vi "Main.vi"() -> ()   [LabVIEW 2019]
uses:
  Controls/Save data file action.ctl
  Sub VIs/_Global variables 1.vi
panel:
  in  "stop":bool
  out "Data file\nInitialization":errorcluster
  out "Statues":string
  out "Boolean":bool
  in  "Initialize":bool
  in  "Recording temperature":enum16{"Sample stage", "Mixing chamber"}(ring)
  in  "Heater control":enum16{"Sample stage", "Mixing chamber"}(ring)
  in  "temp step tolerance":dbl=0.02 format="%_3g"
  in  "temperature step":dbl=0.05 format="%_3g"
  in  "Final temperature":dbl format="%_3g"
  in  "Init temperature":dbl format="%_3g"
  in  "Data acquisition field interval (T)":dbl=0.001
  in  "Current source output":dbl=1e-05
  in  "Starting field":dbl format="%_3g"
  in  "field sweeping rate":dbl=0.02 format="%_3g"
  in  "field adjustment rate":dbl=0.05 format="%_3g"
  in  "Stopping field":dbl format="%_3g"
  out "Current source\nInitialization":errorcluster
  out "Magnet Contro Initialization":errorcluster caption="error out"
  out "Sample temp initialization":errorcluster caption="error out"
  out "Temp control initialization":errorcluster caption="error out"
  in  "Start":bool
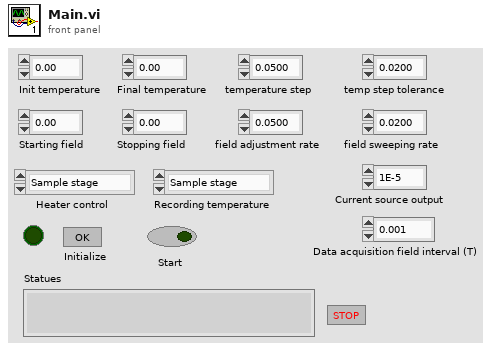
[diagram p1: front panel]
types:
  T1 = typedef "Save data file action.ctl" = enum16{"Create & init file", "Append data", "Close file"}
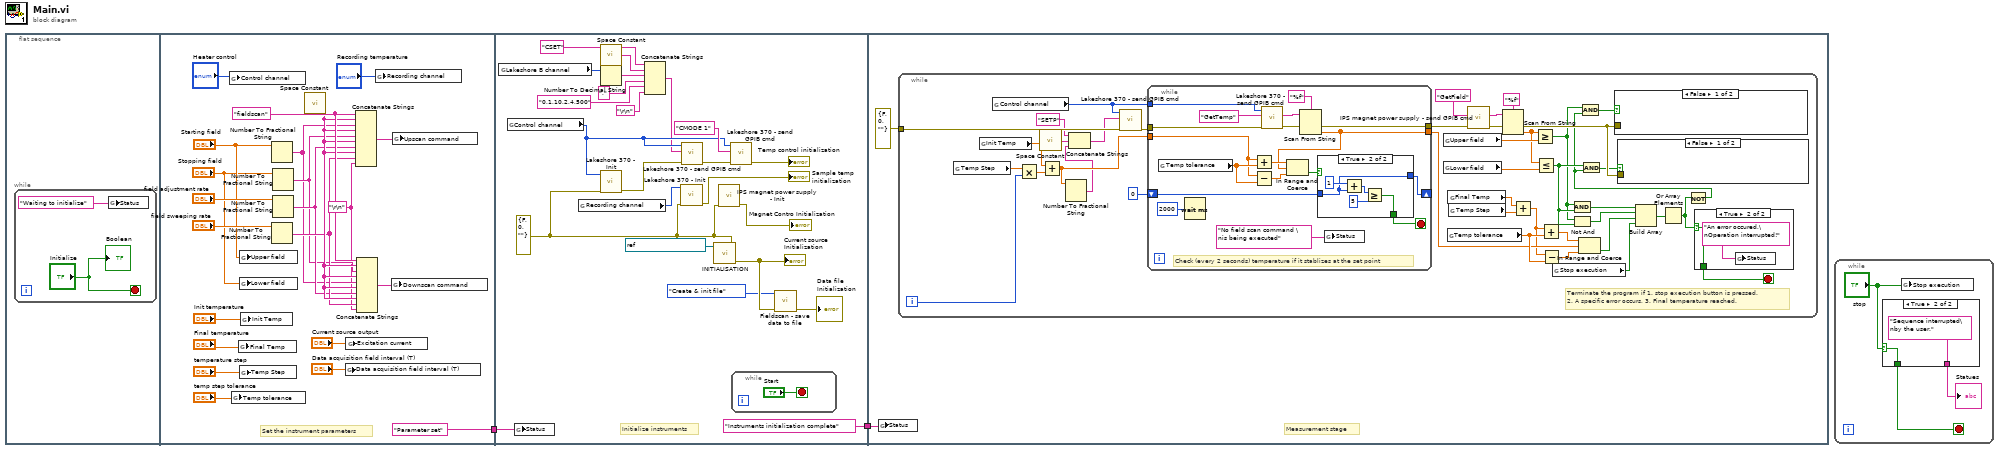
[diagram p0: block diagram]
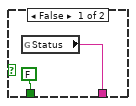
[diagram p2: hidden frame]
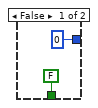
[diagram p4: hidden frame]
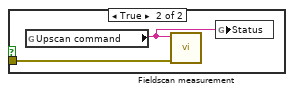
[diagram p5: hidden frame]
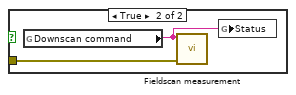
[diagram p6: hidden frame]
diagram:
  n1 = flat-sequence {
    tunnel: ["Parameter set"] -> w2
    tunnel: w2 -> [w43]
    tunnel: ["Instruments initialization complete"] -> w1
    tunnel: w1 -> [w51]
    frame #0 {
      n2 = while {
        stop <- "Initialize" stop-if-true
        n3 = global write "_Global variables 1.vi" "Status"("Waiting to initialize" ("Statues")) -> ()
        "Boolean" <- "Initialize"
      }
    }
    frame #1 {
      w9 = "\r\n"
      w20 = "fieldscan"
      # "Set the instrument parameters"
      n4 = global write "_Global variables 1.vi" "Control channel"("Heater control") -> ()
      n5 = global write "_Global variables 1.vi" "Temp tolerance"("temp step tolerance") -> ()
      n6 = global write "_Global variables 1.vi" "Final Temp"("Final temperature") -> ()
      n7 = global write "_Global variables 1.vi" "Upper field"("Starting field") -> ()
      n8 = global write "_Global variables 1.vi" "Lower field"("Stopping field") -> ()
      n9 = global write "_Global variables 1.vi" "Temp Step"("temperature step") -> ()
      n10 = global write "_Global variables 1.vi" "Init Temp"("Init temperature") -> ()
      n11 = Number To Fractional String(number="Starting field") -> (F-format string=w15:string)  [unwired: 3 in]
      n12 = Number To Fractional String(number="field sweeping rate") -> (F-format string=w18:string)  [unwired: 3 in]
      n13 = Number To Fractional String(number="Stopping field") -> (F-format string=w16:string)  [unwired: 3 in]
      n14 = Number To Fractional String(number="field adjustment rate") -> (F-format string=w17:string)  [unwired: 3 in]
      n15 = call <vilib>:"Space Constant.vi"() -> ("String"=w19:string)
      n16 = global write "_Global variables 1.vi" "Data acquisition field interval (T)"("Data acquisition field interval (T)") -> ()
      n17 = global write "_Global variables 1.vi" "Excitation current"("Current source output") -> ()
      n18 = Concatenate Strings(w20, w19, w15, w19, w16, w19, w17, w19, w18, w9) -> (w10:string)
      n19 = Concatenate Strings(w20, w19, w16, w19, w15, w19, w17, w19, w18, w9) -> (w8:string)
      n20 = global write "_Global variables 1.vi" "Recording channel"("Recording temperature") -> ()
      n21 = global write "_Global variables 1.vi" "Downscan command"(w8) -> ()
      n22 = global write "_Global variables 1.vi" "Upscan command"(w10) -> ()
    }
    frame #2 {
      w46 = errorcluster {"status"=FALSE, "code"=0, "source"=""} ("error in (no error)")
      # "Initialize instruments"
      n23 = global read "_Global variables 1.vi" "Lakeshore B channel"() -> (w34:u8)
      n24 = global read "_Global variables 1.vi" "Control channel"() -> (w35:enum16{"Sample stage", "Mixing chamber"})
      n25 = global write "_Global variables 1.vi" "Status"(w43) -> ()
      n26 = global read "_Global variables 1.vi" "Recording channel"() -> (w44:enum16{"Sample stage", "Mixing chamber"})
      n27 = call <vilib>:"Space Constant.vi"() -> ("String"=w28:string)
      n28 = Number To Decimal String(number=w34) -> (decimal integer string=w32:string)  [unwired: 1 in]
      n29 = call "Lakeshore 370 - Init.vi"("error in (no error)"=w46, "Enum"=w35) -> ("error out"=w45:errorcluster)  [unwired: 8 in, 1 out]
      n30 = Concatenate Strings("CSET" ("Cmd string"), w28, w32, ",", "0,1,10,2,4,500", "\r\n") -> (w29:string)
      n31 = call "Lakeshore 370 - Init.vi"("error in (no error)"=w46, "Enum"=w44) -> ("error out"=→"Sample temp initialization":errorcluster)  [unwired: 8 in, 1 out]
      n32 = call "Lakeshore 370 - send GPIB cmd.vi"("error in (no error)"=w45, "Cmd string"=w29, "Enum"=w35) -> ("error out"=w38:errorcluster)  [unwired: 7 in, 1 out]
      n33 = call "INITIALISATION.vi"("error in (no error)"=w46, "VISAcurrent source"=refnum<visa-resource-name> "GPIB0::12::INSTR" ("Current source")) -> ("error out"=w41:errorcluster)  [unwired: 3 in]
      "Current source\nInitialization" <- w41
      n34 = call "IPS magnet power supply - Init.vi"("error in (no error)"=w46) -> ("error out"=→"Magnet Contro Initialization":errorcluster)  [unwired: 9 in, 1 out]
      n35 = call "Lakeshore 370 - send GPIB cmd.vi"("error in (no error)"=w38, "Cmd string"="CMODE 1", "Enum"=w35) -> ("error out"=→"Temp control initialization":errorcluster)  [unwired: 7 in, 1 out]
      n36 = while {
        stop <- "Start" stop-if-true
      }
      n37 = call "Fieldscan - save data to file.vi"("error in (no error)"=w41, "Action"=Save_data_file_action."Create & init file") -> ("error out"=→"Data file\nInitialization":errorcluster)  [unwired: 8 in, 1 out]
    }
    frame #3 {
      # "Measurement stage"
      n38 = global write "_Global variables 1.vi" "Status"(w51) -> ()
      n39 = while {
        tunnel: errorcluster {"status"=FALSE, "code"=0, "source"=""} ("error in (no error)") -> [w73]
        i -> [w53]
        stop <- w55 stop-if-true
        # "Terminate the program if 1. stop execution button is pressed.\n2. A specific error occurs, 3. Final temperature reached."
        n40 = global read "_Global variables 1.vi" "Temp Step"() -> (w54:dbl)
        n41 = global read "_Global variables 1.vi" "Init Temp"() -> (w71:dbl)
        n42 = global read "_Global variables 1.vi" "Control channel"() -> (w62:enum16{"Sample stage", "Mixing chamber"})
        n43 = Multiply(x=w54, y=w53) -> (x*y=w70:dbl)
        n44 = call <vilib>:"Space Constant.vi"() -> ("String"=w68:string)
        n45 = Add(x=w71, y=w70) -> (x+y=w67:dbl)
        n46 = Number To Fractional String(number=w67) -> (F-format string=w66:string)  [unwired: 3 in]
        n47 = Concatenate Strings("SETP", w68, w66) -> (w65:string)
        n48 = call "Lakeshore 370 - send GPIB cmd.vi"("error in (no error)"=w73, "Cmd string"=w65, "Enum"=w62) -> ("error out"=w72:errorcluster)  [unwired: 7 in, 1 out]
        n49 = while {
          tunnel: w72 -> [w112]
          tunnel: [w107] -> w82
          tunnel: [w105] -> w81
          tunnel: w67 -> [w104]
          shift-right: [w99] -> _
          shift-left: 0 -> [w100]
          tunnel: w62 -> [w98]
          stop <- w101 stop-if-true
          # "Check (every 2 seconds) temperature if it stablizes at the set point"
          n50 = global read "_Global variables 1.vi" "Temp tolerance"() -> (w109:dbl)
          n51 = Wait (ms)(milliseconds to wait=u32 2000) -> ()  [unwired: 1 out]
          n52 = Add(x=w104, y=w109) -> (x+y=w108:dbl)
          n53 = Subtract(x=w104, y=w109) -> (x-y=w110:dbl)
          n54 = call "Lakeshore 370 - send GPIB cmd.vi"("error in (no error)"=w112, "Cmd string"="GetTemp", "Enum"=w98) -> ("error out"=w106:errorcluster, "Response"=w113:string)  [unwired: 7 in]
          n55 = Scan From String(format string="%f", input string=w113, error in=w106) -> (error out=w105:errorcluster, output 1=w107:dbl)  [unwired: 2 in, 2 out]
          n56 = In Range and Coerce(upper limit=w108, x=w107, lower limit=w110) -> (In Range?=w102:bool)  [unwired: 1 out]
          n57 = case shown="True" w102 {
            tunnel: w100 -> [_ w117]
            tunnel: [FALSE w118] -> w101
            tunnel: [0 w117] -> w99
            frame False {
            }
            frame True {
              n58 = Add(x=1, y=w117) -> (x+y=w120:i32)
              n59 = Greater Or Equal?(x=w120, y=5) -> (x >= y?=w118:bool)
            }
          }
          n60 = global write "_Global variables 1.vi" "Status"("No field scan command \nis being executed" ("Downscan command")) -> ()
        }
        n61 = global read "_Global variables 1.vi" "Upper field"() -> (w86:dbl)
        n62 = global read "_Global variables 1.vi" "Lower field"() -> (w84:dbl)
        n63 = global read "_Global variables 1.vi" "Temp tolerance"() -> (w91:dbl)
        n64 = global read "_Global variables 1.vi" "Final Temp"() -> (w75:dbl)
        n65 = global read "_Global variables 1.vi" "Temp Step"() -> (w74:dbl)
        n66 = call "IPS magnet power supply - send GPIB cmd.vi"("error in (no error)"=w81, "Cmd string"="GetField") -> ("error out"=w87:errorcluster, "Response"=w89:string)  [unwired: 8 in]
        n67 = Scan From String(format string="%f", input string=w89, error in=w87) -> (error out=w83:errorcluster, output 1=w85:dbl)  [unwired: 2 in, 2 out]
        n68 = Add(x=w75, y=w74) -> (x+y=w64:dbl)
        n69 = Greater Or Equal?(x=w85, y=w86) -> (x >= y?=w78:bool)
        n70 = Less Or Equal?(x=w85, y=w84) -> (x <= y?=w80:bool)
        n71 = Add(x=w64, y=w91) -> (x+y=w92:dbl)
        n72 = Subtract(x=w64, y=w91) -> (x-y=w93:dbl)
        n73 = global read "_Global variables 1.vi" "Stop execution"() -> (w57:bool)
        n74 = And(x=w78, y=w80) -> (x .and. y?=w61:bool)
        n75 = Not And(1:w80, 2:w78) -> (0:w60:bool)
        n76 = In Range and Coerce(upper limit=w92, x=w82, lower limit=w93) -> (In Range?=w58:bool)  [unwired: 1 out]
        n77 = Build Array(w61, w60, w58, w57) -> (w59:bool[])
        n78 = Or Array Elements(Boolean array=w59) -> (logical OR=w56:bool)
        n79 = Not(x=w56) -> (.not. x?=w77:bool)
        n80 = And(x=w78, y=w77) -> (x .and. y?=w76:bool)
        n81 = And(x=w80, y=w77) -> (x .and. y?=w79:bool)
        n82 = case shown="False" w76 {
          tunnel: w83 -> [_ w125]
          frame False {
          }
          frame True {
            n83 = global read "_Global variables 1.vi" "Downscan command"() -> (w124:string)
            n84 = call "Fieldscan measurement.vi"("error in (no error)"=w125, "Cmd string"=w124) -> ()  [unwired: 9 in, 1 out]
            n85 = global write "_Global variables 1.vi" "Status"(w124) -> ()
          }
        }
        n86 = case shown="False" w79 {
          tunnel: w83 -> [_ w123]
          frame False {
          }
          frame True {
            n87 = global read "_Global variables 1.vi" "Upscan command"() -> (w122:string)
            n88 = call "Fieldscan measurement.vi"("error in (no error)"=w123, "Cmd string"=w122) -> ()  [unwired: 9 in, 1 out]
            n89 = global write "_Global variables 1.vi" "Status"(w122) -> ()
          }
        }
        n90 = case shown="True" w56 {
          selector: w56 -> [w94 w95]
          tunnel: [w94 w95] -> w55
          frame False {
          }
          frame True {
            n91 = global write "_Global variables 1.vi" "Status"("An error occured,\nOperation interrupted!") -> ()
          }
        }
      }
    }
  }
  n92 = while {
    stop <- w128 stop-if-true
    n93 = case shown="True" "stop" {
      selector: "stop" -> [_ w132]
      tunnel: [FALSE w132] -> w128
      tunnel: [w129 "Sequence interrupted\nby the user."] -> w126
      frame False {
        n94 = global read "_Global variables 1.vi" "Status"() -> (w129:string)
      }
      frame True {
      }
    }
    "Statues" <- w126
    n95 = global write "_Global variables 1.vi" "Stop execution"("stop") -> ()
  }
